vi "test123.vi"() -> ()   [LabVIEW 2021]
uses:
  <vilib>/Analysis/Matrix/Datatypes/RealMatrix.ctl
  array -- bilinear regression 2D.ctl
  <vilib>/Analysis/baseanly.llb/Real A x B.vi
  <vilib>/Analysis/Matrix/Numeric/Conversions/Array To Matrix - RA2.vi
  <vilib>/Analysis/Matrix/Numeric/Conversions/Matrix To Array - RM.vi
  <vilib>/Analysis/Matrix/NI_Matrix.lvlib
  <vilib>/Analysis/NI_AALBase.lvlib
panel:
  out "Real 2D Array":dbl[][](array[numeric])
  out "Real Matrix":T1
  out "fit map out":map{T2, dbl}(c390)
  in  "fit":dbl[](array[numeric])=[1.0, 2.0, 3.0, 4.0, 5.0, 6.0]
  out "number of columns tra":i32
  out "number of rows tra":i32
  out "appended array tra":T1
  out "number of columns":i32
  out "number of rows":i32
  out "appended array":T1
  in  "w":dbl[](array[numeric])=[-1.0, 0.0, 1.0, -1.0, 0.0, 1.0, -1.0, 0.0, 1.0]
  in  "y":dbl[](array[numeric])=[-1.0, 0.0, 1.0, -1.0, 0.0, 1.0, -1.0, 0.0, 1.0]
  in  "x":dbl[](array[numeric])=[0.0, 0.0, 0.0, -1.0, -1.0, -1.0, 1.0, 1.0, 1.0]
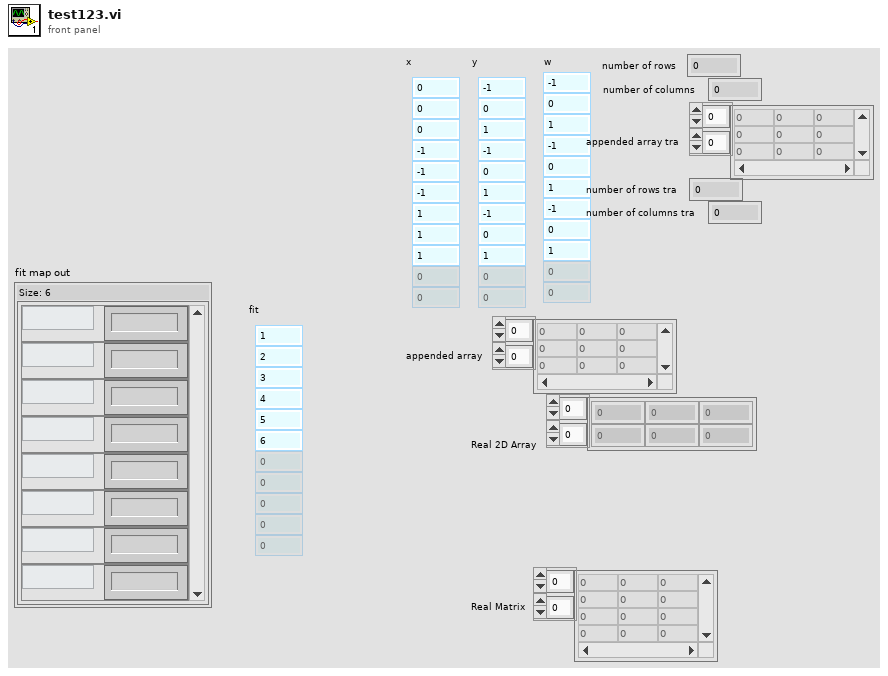
[diagram p1: front panel]
types:
  T1 = typedef "NI_Matrix.lvlib/RealMatrix.ctl" = dbl[][]
  T2 = typedef "array -- bilinear regression 2D.ctl" = enum16{"1", "x", "y", "xx", "xy", "yy", "xxy", "xyy", "yyy", "xxx", "xxyy", "xyyy", "xxxy", "yyyy", "xxxx", "xxz", "xyz", "yyz", "xz", "yz", "z", "wwz", "ywz", "xwz", "xxxw", "xxyw", "xyyw", "yyyw", "xxww", "xyww", "yyww", "xwww", "ywww", "wwww", "ww", "xw", "yw", "w", "wz"}
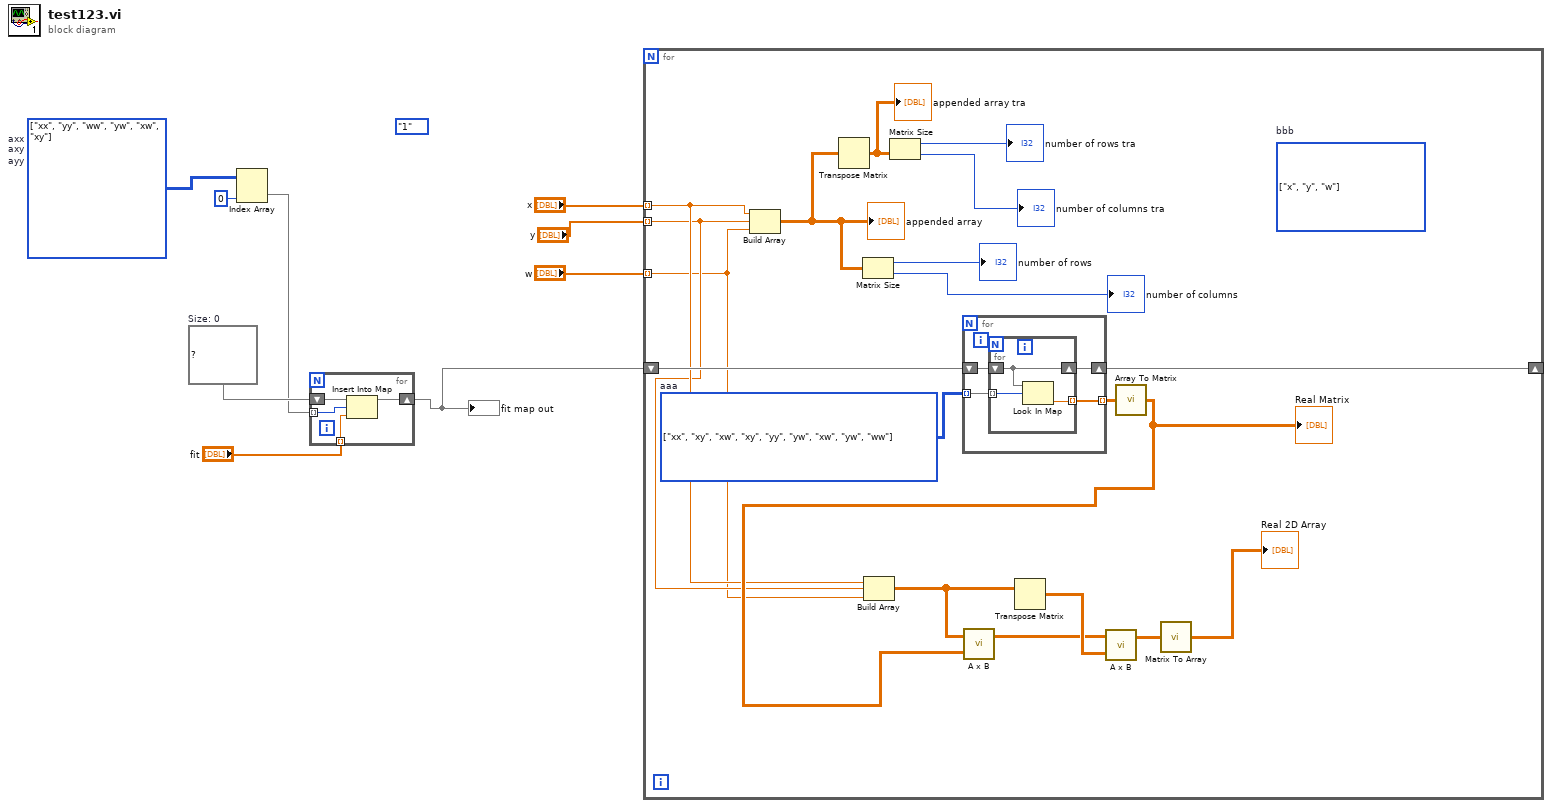
[diagram p0: block diagram]
diagram:
  (unwired) array_--_bilinear_regression_2D."1"
  w6 = map{T2, dbl} {}  # Size: 0
  w4 = T2[][] [[enum."xx"], [enum."yy"], [enum."ww"], [enum."yw"], [enum."xw"], [enum."xy"]] items=["1", "x", "y", "xx", "xy", "yy", "xxy", "xyy", "yyy", "xxx", "xxyy", "xyyy", "xxxy", "yyyy", "xxxx", "xxz", "xyz", "yyz", "xz", "yz", "z", "wwz", "ywz", "xwz", "xxxw", "xxyw", "xyyw", "yyyw", "xxww", "xyww", "yyww", "xwww", "ywww", "wwww", "ww", "xw", "yw", "w", "wz"]  # axx axy ayy
  n1 = Index Array(array=w4, index (col)=0 ("disabled index (col)")) -> (element=w3:T2[])  [unwired: 1 in]
  n2 = for {
    shift-right: [w12] -> w1
    shift-left: w6 -> [w13]
    tunnel: w3 -> [w11] mode=indexing
    tunnel: "fit" -> [w10] mode=indexing
    n3 = Insert Into Map(map in=w13, key=w11, value=w10) -> (map out=w12:map{T2, dbl})  [unwired: 2 out]
  }
  "fit map out" <- w1
  n4 = for {
    tunnel: "x" -> [w17] mode=indexing
    tunnel: "y" -> [w16] mode=indexing
    tunnel: "w" -> [w15] mode=indexing
    shift-right: [w22] -> _
    shift-left: w1 -> [w23]
    (unwired) T2[][] [[enum."x"], [enum."y"], [enum."w"]] items=["1", "x", "y", "xx", "xy", "yy", "xxy", "xyy", "yyy", "xxx", "xxyy", "xyyy", "xxxy", "yyyy", "xxxx", "xxz", "xyz", "yyz", "xz", "yz", "z", "wwz", "ywz", "xwz", "xxxw", "xxyw", "xyyw", "yyyw", "xxww", "xyww", "yyww", "xwww", "ywww", "wwww", "ww", "xw", "yw", "w", "wz"]  # bbb
    w25 = T2[][] [[enum."xx", enum."xy", enum."xw"], [enum."xy", enum."yy", enum."yw"], [enum."xw", enum."yw", enum."ww"]] items=["1", "x", "y", "xx", "xy", "yy", "xxy", "xyy", "yyy", "xxx", "xxyy", "xyyy", "xxxy", "yyyy", "xxxx", "xxz", "xyz", "yyz", "xz", "yz", "z", "wwz", "ywz", "xwz", "xxxw", "xxyw", "xyyw", "yyyw", "xxww", "xyww", "yyww", "xwww", "ywww", "wwww", "ww", "xw", "yw", "w", "wz"]  # aaa
    n5 = Build Array(w17, w16, w15) -> (w30:T1)
    "appended array" <- w30
    n6 = Transpose Matrix(1:w30) -> (0:w27:T1)
    "appended array tra" <- w27
    n7 = Matrix Size(0:w30) -> (1:→"number of rows":i32, 2:→"number of columns":i32)
    n8 = Build Array(w17, w16, w15) -> (w20:T1)
    n9 = Matrix Size(0:w27) -> (1:→"number of rows tra":i32, 2:→"number of columns tra":i32)
    n10 = for {
      tunnel: w25 -> [w36] mode=indexing
      shift-right: [w34] -> w22
      shift-left: w23 -> [w35]
      tunnel: [w33] -> w26 mode=indexing
      n11 = for {
        tunnel: w36 -> [w38] mode=indexing
        shift-right: [w39] -> w34
        shift-left: w35 -> [w39]
        tunnel: [w37] -> w33 mode=indexing
        n12 = Look In Map(map=w39, key=w38) -> (value=w37:dbl)  [unwired: 1 in, 1 out]
      }
    }
    n13 = Transpose Matrix(1:w20) -> (0:w19:T1)
    n14 = call-poly <vilib>:"Array To Matrix.vi"("Real 2D Array"=w26) -> ("Real Matrix"=w24:T1)
    "Real Matrix" <- w24
    n15 = call-poly <vilib>:"A x B.vi"("B"=w24, "A"=w20) -> ("A x B"=w18:T1)  [unwired: 1 out]
    n16 = call-poly <vilib>:"A x B.vi"("B"=w19, "A"=w18) -> ("A x B"=w21:T1)  [unwired: 1 out]
    n17 = call-poly <vilib>:"Matrix To Array.vi"("Real Matrix"=w21) -> ("Real 2D Array"=→"Real 2D Array":dbl[][])
  }
